vi "SpatialSetMagnetometerCorrectionParameters.vi"(0 "error in (no error)":errorcluster, 1 "Correction Parameters":T1, 3 "Device In":u64) -> (7 "error out":errorcluster, 10 "Device Out":u64)   [LabVIEW 2012, in "Phidget Spatial.lvlib"]
doc: "${SetMagnetometerCorrectionParameters:Header}"
uses:
  <instrlib>/Phidgets/Phidget Spatial/Phidget Spatial.lvlib
  <instrlib>/Phidgets/Phidget Common/Phidget Common.lvlib
  phidget22.dll
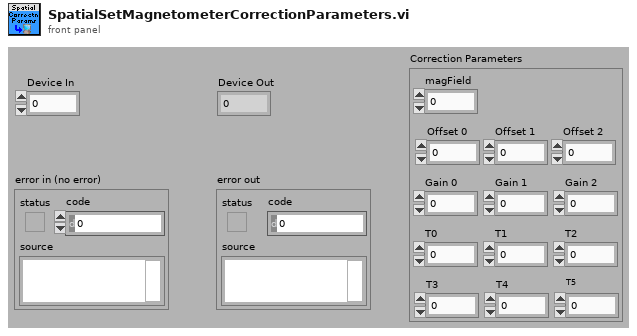
[diagram p1: front panel]
types:
  T1 = cluster{"magField":dbl, "Offset 0":dbl, "Offset 1":dbl, "Offset 2":dbl, "Gain 0":dbl, "Gain 1":dbl, "Gain 2":dbl, "T0":dbl, "T1":dbl, "T2":dbl, "T3":dbl, "T4":dbl, "T5":dbl}
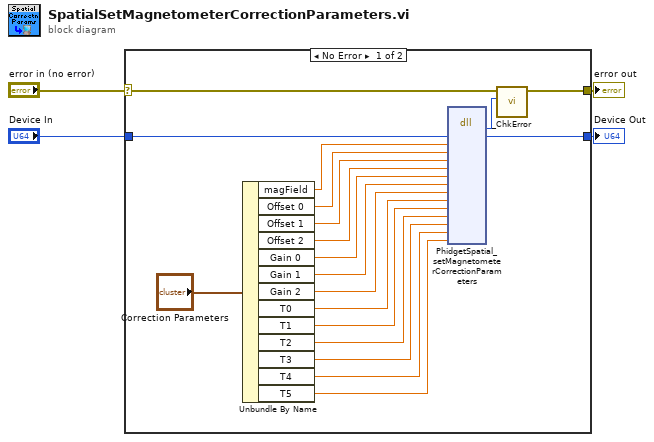
[diagram p0: block diagram]
diagram:
  n1 = case shown="No Error" "error in (no error)" {
    selector: "error in (no error)" -> [w21 w25]
    tunnel: [w20 w25] -> w3
    tunnel: "Device In" -> [w23 w24]
    tunnel: [w22 w24] -> w1
    frame No Error {
      n2 = Unbundle By Name("Correction Parameters") -> ("magField"=w17:dbl, "Offset 0"=w16:dbl, "Offset 1"=w15:dbl, "Offset 2"=w14:dbl, "Gain 0"=w13:dbl, "Gain 1"=w12:dbl, "Gain 2"=w11:dbl, "T0"=w10:dbl, "T1"=w9:dbl, "T2"=w8:dbl, "T3"=w7:dbl, "T4"=w6:dbl, "T5"=w5:dbl)
      n3 = dll-call lib="phidget22.*" fn="PhidgetSpatial_setMagnetometerCorrectionParameters"("phid"=w23, "trigger"=w17, "arg3"=w16, "arg4"=w15, "arg5"=w14, "arg6"=w13, "arg7"=w12, "arg8"=w11, "arg9"=w10, "arg10"=w9, "arg11"=w8, "arg12"=w7, "arg13"=w6, "arg14"=w5) -> ("return type"=w19:i32, "phid"=w22:u64)  [unwired: 16 in, 2 out]
      n4 = call <instrlib>:"_ChkError.vi"("Return Code"=w19, "error in (no error)"=w21) -> ("error out"=w20:errorcluster)  [unwired: 9 in]
    }
    frame Error {
    }
  }
  "error out" <- w3
  "Device Out" <- w1
